vi "C+-math.vi"(9 "S":dbl format="%#_13g", 10 "VMAX":dbl format="%#_13g", 11 "ACC":dbl format="%#_13g") -> (1 "T2":dbl, 2 "T3":dbl, 3 "T1":dbl)   [LabVIEW 2018]
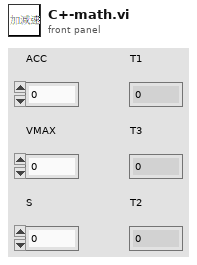
[diagram p1: front panel]
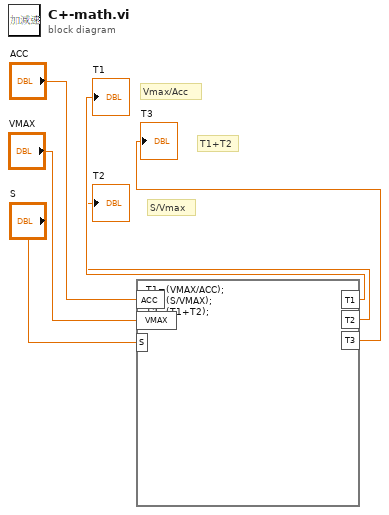
[diagram p0: block diagram]
diagram:
  # "T1+T2"
  # "S/Vmax"
  # "Vmax/Acc"
  n1 = formula code="T1=(VMAX/ACC);\nT2=(S/VMAX);\nT3=(T1+T2);"("ACC"="ACC", "VMAX"="VMAX", "S"="S") -> ("T1"=→"T1":dbl, "T2"=→"T2":dbl, "T3"=→"T3":dbl)
